vi "ProdaNG.CheckProductExists.vi"(8 "error in (no error)":errorcluster, 9 "serialNumber":string, 10 "ID":T3, 11 "dbHandle":i32) -> (0 "error out":errorcluster, 1 "ProcessResult":T1, 2 "ProductID":T2, 3 "dbHandle out":i32, 4 "Results exist?":bool)   [LabVIEW 2016]
doc: "This function returns a product structure for a product, which is identified by a part and a serial number.\nImportant information: The field 'individual' was taken over from the field 'allgemein' of the legacy data directly. Because of this most products have the value 0 further on and only a few the value 1. \nParameter:\nhandle is an Integer, which is returned by the function Login() at the creation of a new connection.\nwabcoPartId is the Id of the part.\nserialNumber is the serial number of the product for the part above.\nproduct is a pointer on a product structure, which is filled if the returncode is 0. The structure must be defined in the calling program.\n\nReturncodes:\n0 No error\n< 0 ORACLE Error code\n6 (ERROR_INVALID_HANDLE) in case of an invalid handle\n1403 Record does not exist"
uses:
  Controls/ProdaNG.Identification.ctl
  Controls/ProdaNG.Product.ctl
  Controls/ProdaNG.ProcessResult.ctl
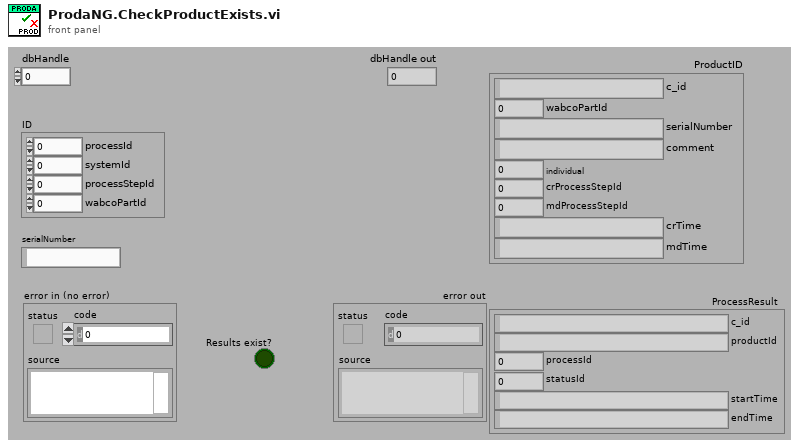
[diagram p1: front panel]
types:
  T1 = typedef "ProdaNG.ProcessResult.ctl" = cluster{"c_id":string, "productId":string, "processId":i32, "statusId":i32, "startTime":string, "endTime":string}
  T2 = typedef "ProdaNG.Product.ctl" = cluster{"c_id":string, "wabcoPartId":i32, "serialNumber":string, "comment":string, "individual":i32, "crProcessStepId":i32, "mdProcessStepId":i32, "crTime":string, "mdTime":string}
  T3 = typedef "ProdaNG.Identification.ctl" = cluster{"processId":i32, "systemId":i32, "processStepId":i32, "wabcoPartId":i32}
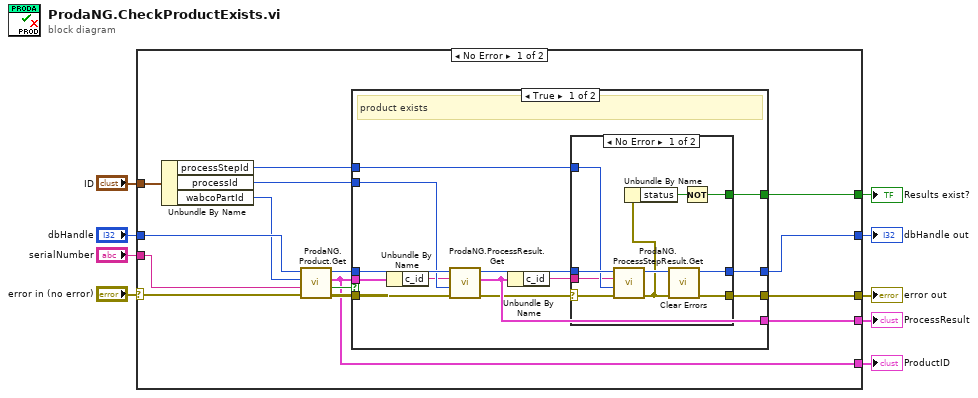
[diagram p0: block diagram]
diagram:
  n1 = case shown="No Error" "error in (no error)" {
    selector: "error in (no error)" -> [w24 w52]
    tunnel: [w10 w52] -> w8
    tunnel: "dbHandle" -> [w21 w51]
    tunnel: [w12 w51] -> w6
    tunnel: "serialNumber" -> [w18 _]
    tunnel: "ID" -> [w20 _]
    tunnel: [w17 _] -> w3
    tunnel: [w13 _] -> w2
    tunnel: [w11 _] -> w1
    frame No Error {
      n2 = Unbundle By Name(w20) -> ("processStepId"=w14:i32, "processId"=w15:i32, "wabcoPartId"=w19:i32)
      n3 = call "ProdaNG.Product.Get.vi"("error in (no error)"=w24, "serialNumber"=w18, "wabcoPartId"=w19, "dbHandle"=w21) -> ("error out"=w23:errorcluster, "found"=w22:bool, "Product"=w13:T2, "dbHandle out"=w16:i32)  [unwired: 4 in]
      n4 = case shown="True" w22 {
        tunnel: w23 -> [w36 w50]
        tunnel: [w33 w50] -> w10
        tunnel: [w25 _] -> w17
        tunnel: w16 -> [w35 w49]
        tunnel: [w34 w49] -> w12
        tunnel: w15 -> [w30 _]
        tunnel: w14 -> [w31 _]
        tunnel: w13 -> [w32 _]
        tunnel: [w27 _] -> w11
        frame True {
          # "product exists"
          n5 = Unbundle By Name(w32) -> ("c_id"=w29:string)
          n6 = call "ProdaNG.ProcessResult.Get.vi"("error in (no error)"=w36, "processId"=w30, "productId"=w29, "dbHandle"=w35) -> ("error out"=w26:errorcluster, "ProcessResult"=w27:T1, "dbHandle out"=w37:i32)  [unwired: 4 in, 1 out]
          n7 = Unbundle By Name(w27) -> ("c_id"=w28:string)
          n8 = case shown="No Error" w26 {
            selector: w26 -> [w41 w48]
            tunnel: w37 -> [w46 w47]
            tunnel: [w45 w47] -> w34
            tunnel: [w42 w48] -> w33
            tunnel: w31 -> [w44 _]
            tunnel: w28 -> [w43 _]
            tunnel: [w38 _] -> w25
            frame No Error {
              n9 = call "ProdaNG.ProcessStepResult.Get.vi"("error in (no error)"=w41, "processStepId"=w44, "processResultId"=w43, "dbHandle"=w46) -> ("error out"=w39:errorcluster, "dbHandle out"=w45:i32)  [unwired: 4 in, 2 out]
              n10 = Unbundle By Name(w39) -> ("status"=w40:bool)
              n11 = call <vilib>:"Clear Errors.vi"("error in (no error)"=w39) -> ("error out"=w42:errorcluster)  [unwired: 5 in, 1 out]
              n12 = Not(x=w40) -> (.not. x?=w38:bool)
            }
            frame Error {
            }
          }
        }
        frame False {
          # "product missing"
        }
      }
    }
    frame Error {
    }
  }
  "error out" <- w8
  "dbHandle out" <- w6
  "Results exist?" <- w3
  "ProductID" <- w2
  "ProcessResult" <- w1
